vi "ReadLightTower&SwitchStatus.vi"(6 "Accessors:ValuesToSet(OID_TYPE)":string[][](array[string]), 7 "IP Address of SNMP Device":string, 8 "error in (no error)":errorcluster, 9 "Timeout(ms)":i32, 10 "Community Name":string, 11 "UDP Network Connection in":refnum<k16>) -> (0 "error out":errorcluster, 3 "Light Tower":T1)   [LabVIEW 2018, in "SensorPlugins.lvlib" / "RoomAlert.lvclass"]
doc: "Reads the Light Tower and Switch Sensor status"
uses:
  RoomAlert.lvclass
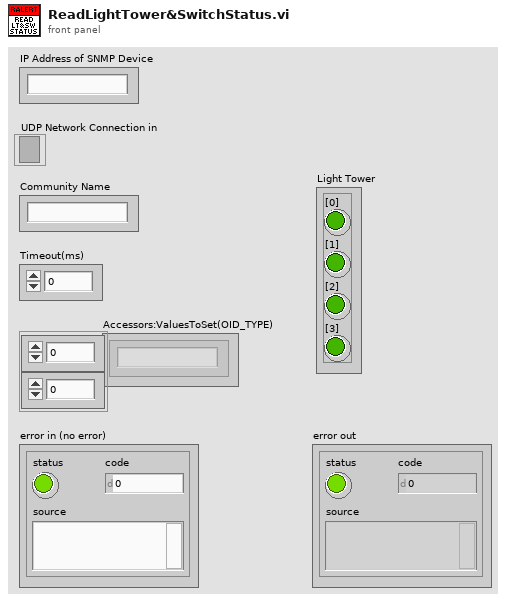
[diagram p1: front panel]
types:
  T1 = cluster{"[0]":bool, "[1]":bool, "[2]":bool, "[3]":bool}
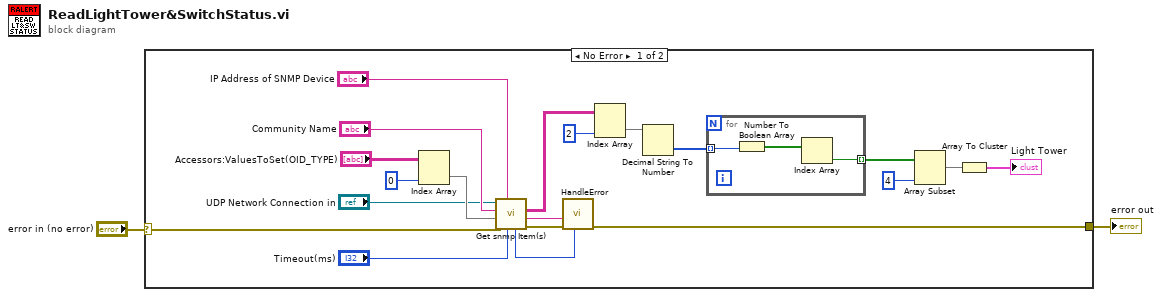
[diagram p0: block diagram]
diagram:
  n1 = case shown="No Error" "error in (no error)" {
    selector: "error in (no error)" -> [w4 w26]
    tunnel: [w3 w26] -> w1
    frame No Error {
      n2 = Index Array(array="Accessors:ValuesToSet(OID_TYPE)", index (col)=0 ("disabled index (col)")) -> (element=w16:string[])  [unwired: 1 in]
      n3 = call "Get snmp Item(s).vi"("timeout ms (25000)"="Timeout(ms)", "IP Address of SNMP Device"="IP Address of SNMP Device", "error in (no error)"=w4, "OID ARRAY"=w16, "Community Name"="Community Name", "connection ID in"="UDP Network Connection in") -> ("error out"=w19:errorcluster, "error-string"=w21:string, "SnmpDataAsStrings"=w12:string[][], "error-status"=w22:u8)  [unwired: 1 in, 1 out]
      n4 = call "HandleError.vi"("error-status"=w22, "Error In"=w19, "Error String"=w21) -> ("Error Out"=w3:errorcluster)  [unwired: 8 in]
      n5 = Index Array(array=w12, index (col)=2 ("disabled index (col)")) -> (element=w10:string[])  [unwired: 1 in]
      n6 = Decimal String To Number(string=w10) -> (number=w9:i32[])  [unwired: 2 in, 1 out]
      n7 = for {
        tunnel: w9 -> [w24] mode=indexing
        tunnel: [w23] -> w8 mode=indexing
        n8 = Number To Boolean Array(number=w24) -> (Boolean array=w25:bool[])
        n9 = Index Array(array=w25) -> (element=w23:bool)  [unwired: 1 in]
      }
      n10 = Array Subset(array=w8, length=4) -> (w6:bool[])  [unwired: 1 in]
      n11 = Array To Cluster(array=w6) -> (cluster=→"Light Tower":T1)
    }
    frame Error {
    }
  }
  "error out" <- w1
